vi "Host.vi"() -> ()   [LabVIEW 2025]
uses:
  <vilib>/FPGAPlugInAG/cRIO-9035/niLvFpga_Open_cRIO-9035.vi
  <vilib>/rvi/interface/common/dynamic/niFpgaDynamicAddResources.vi
  <vilib>/FPGAPlugInAG/Dynamic/niLvFpga_Reset_Dynamic.vi
  <vilib>/Utility/error.llb/Error Cluster From Error Code.vi
  <vilib>/rvi/errors/niLvFpgaAdjustHostInterfaceError.vi
  <vilib>/FPGAPlugInAG/Dynamic/niLvFpga_Run_Dynamic.vi
  <vilib>/FPGAPlugInAG/Dynamic/niLvFpga_Close_Dynamic.vi
  <vilib>/rvi/interface/nirviOpenFPGA/nirviOpenFPGA.xnode
  FPGA Bitfiles/hmmlponfpgav1_FPGATarget_Target_idKjxc95-ds.lvbitx
  Target.vi
  <vilib>/rvi/interface/nirviMethod/nirviMethod.xnode
  <vilib>/rvi/interface/nirviCloseFPGA/nirviCloseFPGA.xnode
  <vilib>/rvi/errors/niLvFpgaMergeErrorWithErrorCode.vi
  <vilib>/FPGAPlugInAG/Dynamic/niLvFpga_WriteFifo_Dynamic.vi
  <vilib>/FPGAPlugInAG/Dynamic/niLvFpga_ReadFifo_Dynamic.vi
panel:
  out "output array":sgl[](array[numeric])
  out "input":dbl[][](array[numeric])
  out "size(s) 2":i32
  out "size(s)":i32[](array[numeric])
  out "Uncontrolled Acceleration":dynamicdata(graph)
  out "Control Force":sgl[](graph)
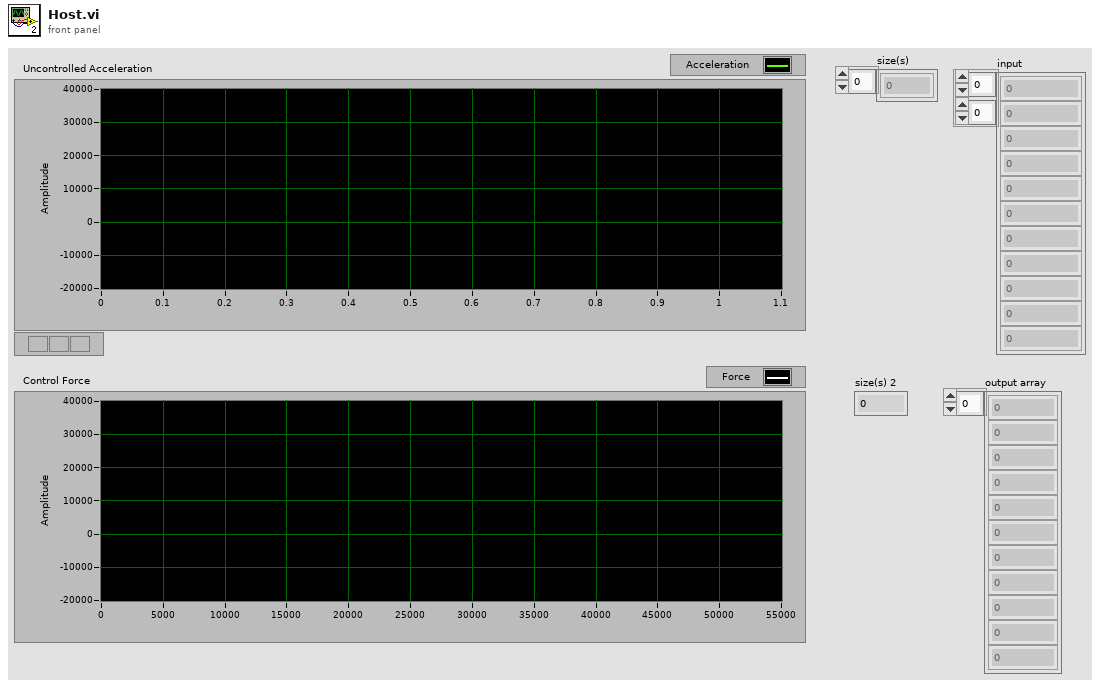
[diagram p1: front panel]
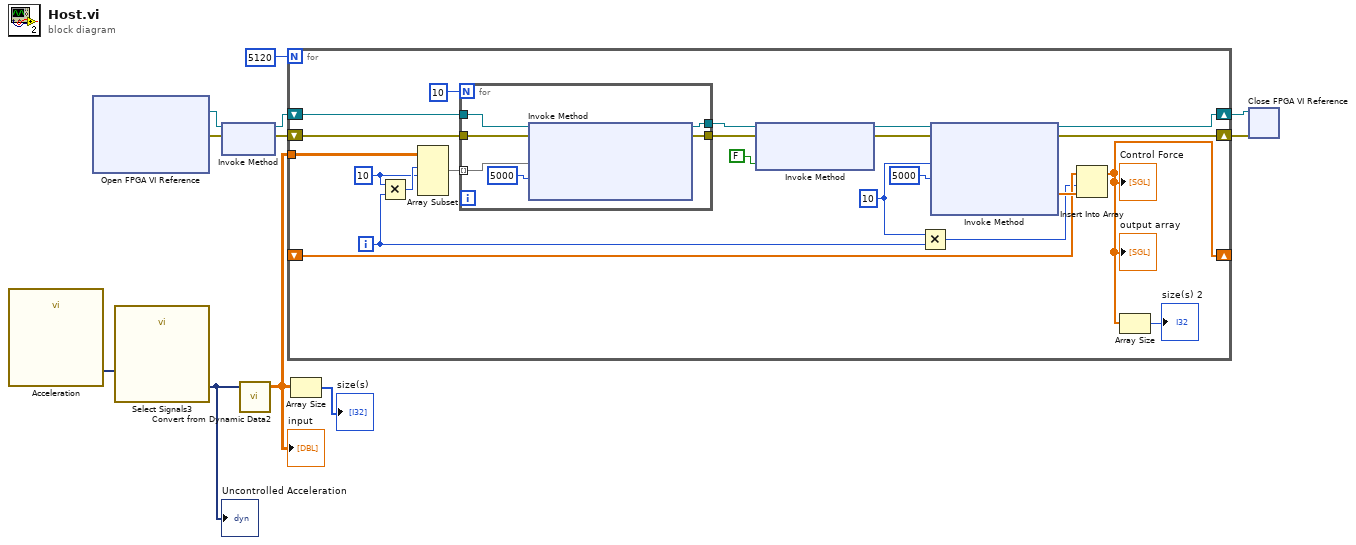
[diagram p0: block diagram]
diagram:
  n1 = call "Acceleration"() -> ("Signals"=w11:dynamicdata)  [unwired: 6 in, 5 out]
  n2 = xnode "Open FPGA VI Reference"() -> ("FPGA VI Reference Out"=w10:refnum<k20>, "error out"=w7:errorcluster)  [unwired: 2 in]
  n3 = call "Select Signals3"("Signals"=w11) -> ("Signal Out"=w6:dynamicdata)  [unwired: 9 in, 1 out]
  "Uncontrolled Acceleration" <- w6
  n4 = xnode "Invoke Method"("FPGA VI Reference In"=w10, "error in"=w7) -> ("FPGA VI Reference Out"=w9:refnum<k20>, "error out"=w8:errorcluster)
  n5 = call "Convert from Dynamic Data2"("Dynamic Data Type"=w6) -> ("Array"=w1:dbl[][])  [unwired: 3 in]
  "input" <- w1
  n6 = for {
    N: 5120 -> [_]
    shift-right: [w27] -> w4
    shift-left: w9 -> [w33]
    shift-right: [w26] -> w3
    shift-left: w8 -> [w32]
    shift-right: [w20] -> _
    shift-left: _ -> [w19]
    tunnel: w1 -> [w13]
    i -> [w15]
    w14 = 10 ("length")
    w18 = u32 10 ("Number of Elements")
    n7 = Multiply(x=w14, y=w15) -> (x*y=w16:i32)
    n8 = Array Subset(array=w13, index (row)=w16, length (row)=w14) -> (w12:dbl[][])  [unwired: 2 in]
    n9 = for {
      N: 10 -> [_]
      tunnel: w33 -> [w39]
      tunnel: w32 -> [w38]
      tunnel: [w36] -> w25
      tunnel: [w35] -> w24
      tunnel: w12 -> [w34] mode=indexing
      n10 = xnode "Invoke Method"("FPGA VI Reference In"=w39, "error in"=w38, "Data"=w34, "Timeout (ms)"=5000) -> ("FPGA VI Reference Out"=w36:refnum<k20>, "error out"=w35:errorcluster)  [unwired: 1 out]
    }
    n11 = xnode "Invoke Method"("FPGA VI Reference In"=w25, "error in"=w24, "Wait Until Done (F)"=FALSE) -> ("FPGA VI Reference Out"=w30:refnum<k20>, "error out"=w29:errorcluster)
    n12 = Multiply(x=w18, y=w15) -> (x*y=w17:u32)
    n13 = xnode "Invoke Method"("FPGA VI Reference In"=w30, "error in"=w29, "Number of Elements"=w18, "Timeout (ms)"=5000) -> ("FPGA VI Reference Out"=w27:refnum<k20>, "error out"=w26:errorcluster, "Data"=w21:sgl[])  [unwired: 1 out]
    n14 = Insert Into Array(array=w19, index=w17, new element=w21) -> (w20:sgl[])
    "Control Force" <- w20
    "output array" <- w20
    n15 = Array Size(array=w20) -> (size(s)=→"size(s) 2":i32)
  }
  n16 = Array Size(array=w1) -> (size(s)=→"size(s)":i32[])
  n17 = xnode "Close FPGA VI Reference"("FPGA VI Reference In"=w4, "error in"=w3) -> ()  [unwired: 1 out]
